vi "Write Times Repeat.vi"(8 "error in (no error)":errorcluster, 10 "Times Repeat":u32=1 min=1 step=1, 11 "RepeatingDirector in":refnum<class "RepeatingDirector.lvclass">) -> (0 "error out":errorcluster, 3 "RepeatingDirector out":refnum<class "RepeatingDirector.lvclass">)   [LabVIEW 2023, in "HAF.lvlib" / "RepeatingDirector.lvclass"]
doc: "Stores the number of times the Commands should be repeated."
uses:
  RepeatingDirector.lvclass
  RepeatingDirector.lvclass/RepeatingDirector.ctl
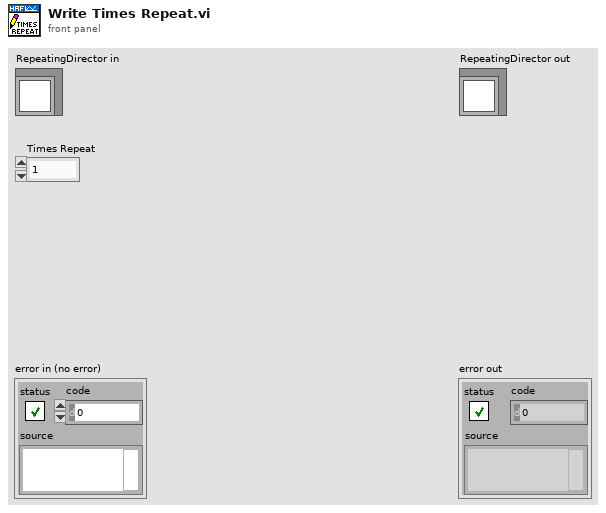
[diagram p1: front panel]
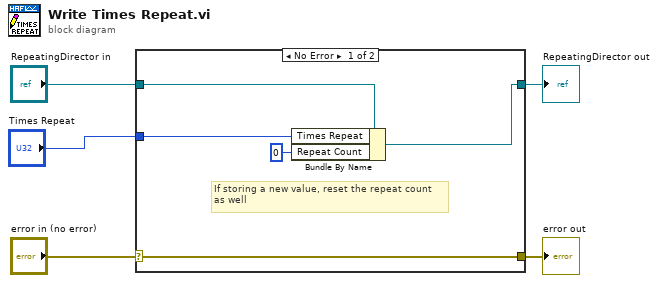
[diagram p0: block diagram]
diagram:
  n1 = case shown="No Error" "error in (no error)" {
    selector: "error in (no error)" -> [w10 w11]
    tunnel: [w10 w11] -> w4
    tunnel: [w8 w12] -> w2
    tunnel: "RepeatingDirector in" -> [w9 w12]
    tunnel: "Times Repeat" -> [w7 _]
    frame No Error {
      # "If storing a new value, reset the repeat count\nas well"
      n2 = Bundle By Name(cluster=w9, "Times Repeat"=w7, "Repeat Count"=u32 0) -> (w8:refnum<class "RepeatingDirector.lvclass">)
    }
    frame Error {
    }
  }
  "error out" <- w4
  "RepeatingDirector out" <- w2
